vi "VI Tree.vi"   [LabVIEW 2020, in "Agilent 34405.lvlib"]
doc: "This is the instrument driver for the Agilent 34405A and 34450A. The VI Tree displays all the user-callable VIs of the instrument driver in an organized table."
uses:
  <instrlib>/Agilent 34405/Agilent 34405.lvlib
panel:
  # "(c) 2009 - 2015 National Instruments Corporation.  ALL RIGHTS RESERVED."
  # "SEE DIAGRAM\nFOR VI TREE."
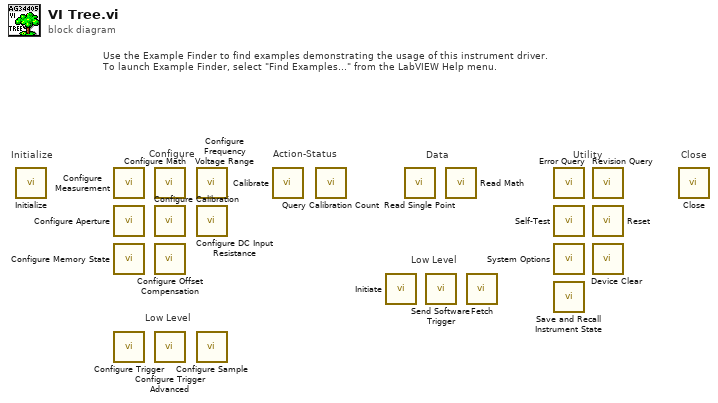
[diagram p0: block diagram]
diagram:
  # "Action-Status"
  # "Use the Example Finder to find examples demonstrating the usage of this instrument driver.\nTo launch Example Finder, select \"Find Examples...\" from the LabVIEW Help menu."
  # "Low Level"
  # "Low Level"
  # "Configure"
  # "Utility"
  # "Data"
  # "Close"
  # "Initialize"
  n1 = call <instrlib>:"Initialize.vi"() -> ()  [unwired: 9 in, 3 out]
  n2 = call <instrlib>:"Configure Measurement.vi"() -> ()  [unwired: 10 in, 2 out]
  n3 = call <instrlib>:"Configure Aperture.vi"() -> ()  [unwired: 10 in, 2 out]
  n4 = call <instrlib>:"Configure Memory State.vi"() -> ()  [unwired: 10 in, 2 out]
  n5 = call <instrlib>:"Configure Trigger.vi"() -> ()  [unwired: 10 in, 2 out]
  n6 = call <instrlib>:"Configure Math.vi"() -> ()  [unwired: 14 in, 2 out]
  n7 = call <instrlib>:"Configure Calibration.vi"() -> ()  [unwired: 10 in, 2 out]
  n8 = call <instrlib>:"Configure Offset Compensation.vi"() -> ()  [unwired: 10 in, 2 out]
  n9 = call <instrlib>:"Configure Trigger Advanced.vi"() -> ()  [unwired: 10 in, 2 out]
  n10 = call <instrlib>:"Configure Frequency Voltage Range.vi"() -> ()  [unwired: 10 in, 2 out]
  n11 = call <instrlib>:"Configure DC Input Resistance.vi"() -> ()  [unwired: 10 in, 2 out]
  n12 = call <instrlib>:"Configure Sample.vi"() -> ()  [unwired: 10 in, 2 out]
  n13 = call <instrlib>:"Calibrate.vi"() -> ()  [unwired: 9 in, 3 out]
  n14 = call <instrlib>:"Query Calibration Count.vi"() -> ()  [unwired: 9 in, 3 out]
  n15 = call <instrlib>:"Initiate.vi"() -> ()  [unwired: 10 in, 2 out]
  n16 = call <instrlib>:"Read Single Point.vi"() -> ()  [unwired: 9 in, 3 out]
  n17 = call <instrlib>:"Send Software Trigger.vi"() -> ()  [unwired: 10 in, 2 out]
  n18 = call <instrlib>:"Read Math.vi"() -> ()  [unwired: 6 in, 6 out]
  n19 = call <instrlib>:"Fetch.vi"() -> ()  [unwired: 9 in, 3 out]
  n20 = call <instrlib>:"Error Query.vi"() -> ()  [unwired: 8 in, 4 out]
  n21 = call <instrlib>:"Self-Test.vi"() -> ()  [unwired: 8 in, 4 out]
  n22 = call <instrlib>:"System Options.vi"() -> ()  [unwired: 10 in, 2 out]
  n23 = call <instrlib>:"Save and Recall Instrument State.vi"() -> ()  [unwired: 10 in, 2 out]
  n24 = call <instrlib>:"Revision Query.vi"() -> ()  [unwired: 8 in, 4 out]
  n25 = call <instrlib>:"Reset.vi"() -> ()  [unwired: 10 in, 2 out]
  n26 = call <instrlib>:"Device Clear.vi"() -> ()  [unwired: 10 in, 2 out]
  n27 = call <instrlib>:"Close.vi"() -> ()  [unwired: 11 in, 1 out]
